vi "stations PING check client.vi"(4 "error in (no error)":errorcluster, 6 "Timeout, ms (10000)":i32=10000, 7 "Client IP (\"\")":string) -> (0 "error out":errorcluster, 2 "TestStation Client?":bool, 3 "Response":string)   [LabVIEW 2011]
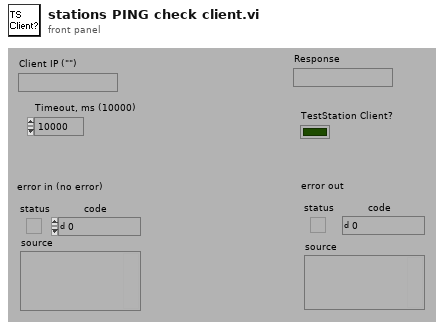
[diagram p1: front panel]
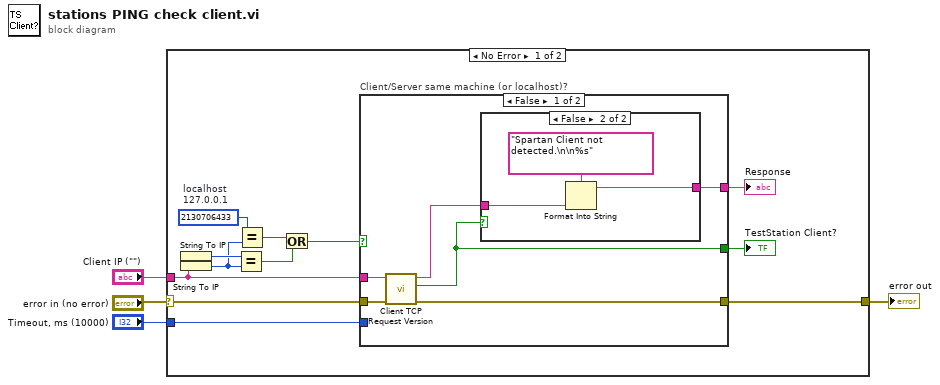
[diagram p0: block diagram]
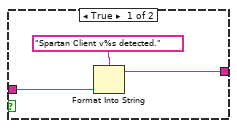
[diagram p2: hidden frame]
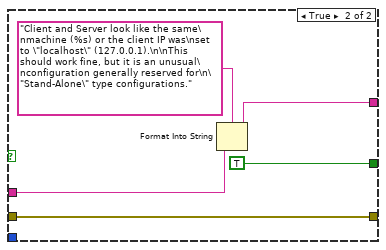
[diagram p3: hidden frame]
diagram:
  n1 = case shown="No Error" "error in (no error)" {
    selector: "error in (no error)" -> [w13 w34]
    tunnel: "Timeout, ms (10000)" -> [w16 _]
    tunnel: "Client IP (\"\")" -> [w11 _]
    tunnel: [w14 w34] -> w2
    frame No Error {
      w7 = u32 2130706433  # localhost 127.0.0.1
      n2 = String To IP() -> (0:w10:u32)  [unwired: 1 out]
      n3 = String To IP(1:w11) -> (0:w8:u32)
      n4 = Equal?(x=w10, y=w8) -> (x = y?=w9:bool)
      n5 = Equal?(x=w7, y=w8) -> (x = y?=w6:bool)
      n6 = Or(x=w6, y=w9) -> (x .or. y?=w5:bool)
      n7 = case "Client/Server same machine (or localhost)?" shown="False" w5 {
        tunnel: w16 -> [_ _]
        tunnel: [w21 w29] -> w15
        tunnel: [w22 w32] -> w14
        tunnel: w13 -> [w19 w32]
        tunnel: [w17 TRUE] -> w12
        tunnel: w11 -> [w20 w30]
        frame False {
          n8 = call "Client TCP Request Version.vi"("error in (no error)"=w19, "Client IP"=w20) -> ("error out"=w22:errorcluster, "Client Detected?"=w17:bool, "Client Version String"=w18:string)  [unwired: 7 out]
          n9 = case shown="False" w17 {
            tunnel: [w25 w28] -> w21
            tunnel: w18 -> [w23 w26]
            frame True {
              n10 = Format Into String(format string="Spartan Client v%s detected.", w23) -> (resulting string=w25:string)  [unwired: 2 in, 1 out]
            }
            frame False {
              n11 = Format Into String(format string="Spartan Client not detected.\n\n%s", w26) -> (resulting string=w28:string)  [unwired: 2 in, 1 out]
            }
          }
        }
        frame True {
          n12 = Format Into String(format string="Client and Server look like the same\nmachine (%s) or the client IP was\nset to \"localhost\" (127.0.0.1).\n\nThis should work fine, but it is an unusual\nconfiguration generally reserved for\n\"Stand-Alone\" type configurations.", w30) -> (resulting string=w29:string)  [unwired: 2 in, 1 out]
        }
      }
      "Response" <- w15
      "TestStation Client?" <- w12
    }
    frame Error {
    }
  }
  "error out" <- w2
